vi "Store Static VI References for Subpanel.vi"(8 "error in (no error)":errorcluster, 11 "DAQ Configuration in":refnum<class "DAQ Configuration.lvclass">) -> (0 "error out":errorcluster, 3 "DAQ Configuration out":refnum<class "DAQ Configuration.lvclass">)   [LabVIEW 2016, in "Hardware.lvlib" / "DAQ Configuration.lvclass"]
uses:
  DAQ Configuration.lvclass
  C:/Program Files (x86)/National Instruments/LabVIEW 2016/user.lib/Configuration Dialog Actor/Configuration.lvclass
  HW Config/HW Configuration.vi
  <userlib>/Configuration Dialog Actor/Configuration.lvclass
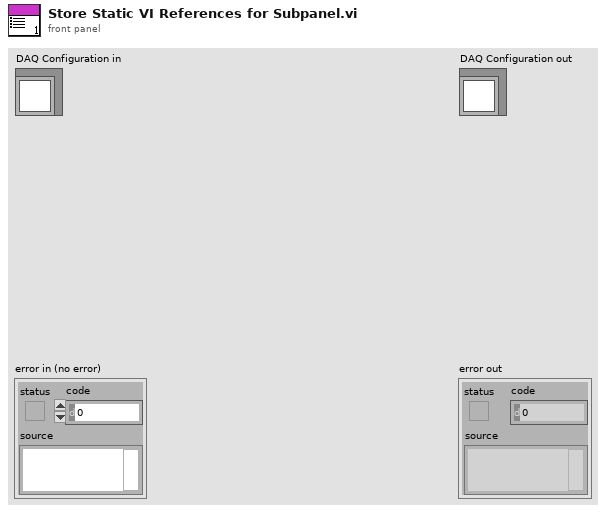
[diagram p1: front panel]
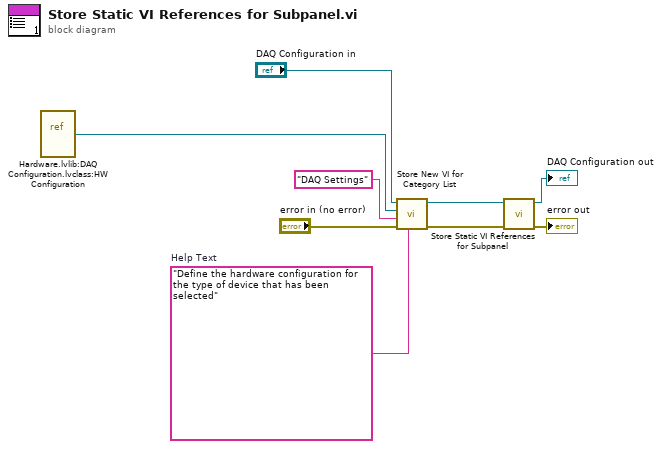
[diagram p0: block diagram]
diagram:
  w2 = "Define the hardware configuration for the type of device that has been selected"  # Help Text
  n1 = vi-ref "Hardware.lvlib:DAQ Configuration.lvclass:HW Configuration.vi"() -> (w3:refnum<vi>)
  n2 = call <userlib>:"Store New VI for Category List.vi"("Help Text"=w2, "error in (no error)"="error in (no error)", "String"="DAQ Settings", "VI Refnum"=w3, "Configuration in"="DAQ Configuration in") -> ("error out"=w4:errorcluster, "Configuration out"=w6:refnum<class "DAQ Configuration.lvclass">)  [unwired: 5 in]
  n3 = call-parent "Store Static VI References for Subpanel.vi"("error in (no error)"=w4, "Configuration in"=w6) -> ("error out"=→"error out":errorcluster, "Configuration out"=→"DAQ Configuration out":refnum<class "DAQ Configuration.lvclass">)  [unwired: 8 in]
